vi "AutoFindRepoPath.vi"(8 "error in (no error)":errorcluster) -> (0 "error out":errorcluster, 3 "Repo Path":path)   [LabVIEW 2019, in "Hawkeye.lvlib"]
uses:
  Hawkeye.lvlib
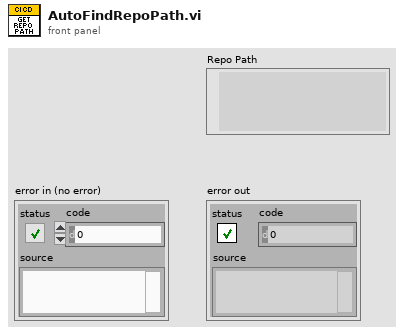
[diagram p1: front panel]
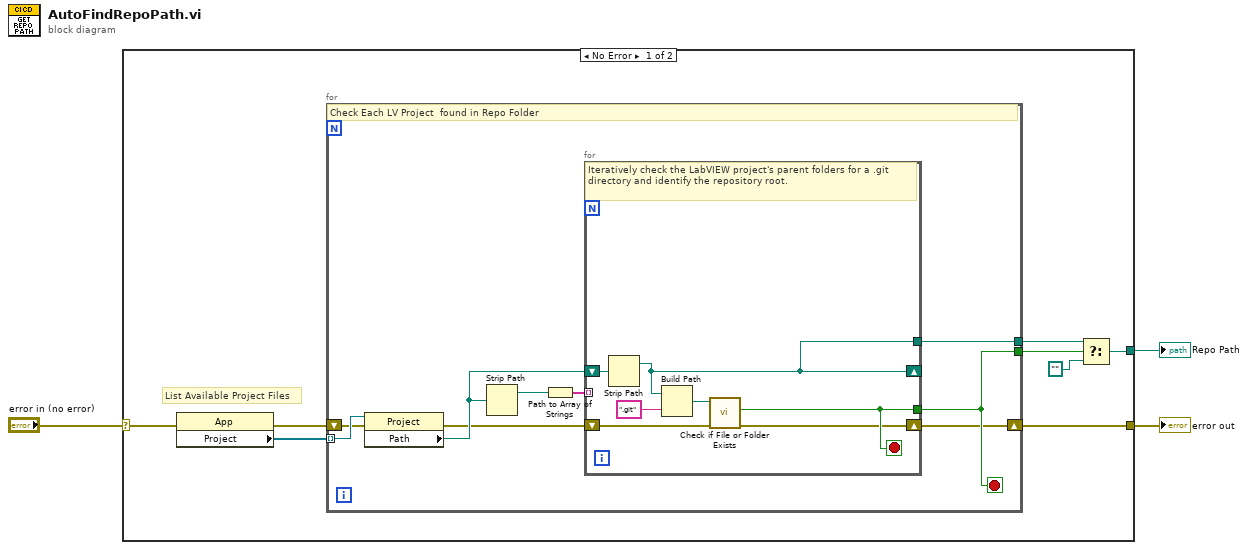
[diagram p0: block diagram]
diagram:
  n1 = case shown="No Error" "error in (no error)" {
    selector: "error in (no error)" -> [w4 w28]
    tunnel: [w7 _] -> w3
    tunnel: [w5 w28] -> w2
    frame No Error {
      # "List Available Project Files"
      n2 = property class="App"(error in=w4) -> (error out=w10:errorcluster, "Project"=w11:refnum<vi>[])  [unwired: 1 in, 1 out]
      n3 = for {
        tunnel: w11 -> [w20] mode=indexing
        tunnel: [w18] -> w8
        tunnel: [w13] -> w9
        shift-right: [w12] -> w5
        shift-left: w10 -> [w14]
        stop <- w13 stop-if-true
        # "Check Each LV Project  found in Repo Folder"
        n4 = property class="Project"(reference=w20, error in=w14) -> (error out=w15:errorcluster, "Path"=w17:path)  [unwired: 1 out]
        n5 = Strip Path(path=w17) -> (stripped path=w16:path)  [unwired: 1 out]
        n6 = Path to Array of Strings(0:w16) -> (2:w19:string[])  [unwired: 1 out]
        n7 = for {
          tunnel: w19 -> [_] mode=indexing
          shift-right: [w24] -> _
          shift-left: w17 -> [w27]
          tunnel: [w24] -> w18
          tunnel: [w23] -> w13
          shift-right: [w21] -> w12
          shift-left: w15 -> [w22]
          stop <- w23 stop-if-true
          # "Iteratively check the LabVIEW project's parent folders for a .git directory and identify the repository root."
          n8 = Strip Path(path=w27) -> (stripped path=w24:path)  [unwired: 1 out]
          n9 = Build Path(base path=w24, name or relative path=".git") -> (appended path=w25:path)
          n10 = call <vilib>:"Check if File or Folder Exists.vi"("error in (no error)"=w22, "path"=w25) -> ("error out"=w21:errorcluster, "file or folder exists?"=w23:bool)  [unwired: 7 in, 1 out]
        }
      }
      n11 = Select(t=w8, s=w9, f=path "") -> (s? t:f=w7:path)
    }
    frame Error {
    }
  }
  "Repo Path" <- w3
  "error out" <- w2
